vi "get channels.vi"(11 "EthernetIP configuration in":refnum<class "EIP Tags Configuration.lvclass">) -> (2 "channels":refnum<class "TBM channel.lvclass">[](array[class]), 3 "EthernetIP configuration out":refnum<class "EIP Tags Configuration.lvclass">)   [LabVIEW 2013, in "EIP Tags Configuration.lvclass"]
uses:
  EIP Tags Configuration.lvclass
  <vilib>/NI/Tag Bus Module Framework/channel/TBM channel.lvclass
  EIP Tags Configuration.lvclass/EIP Tags Configuration.ctl
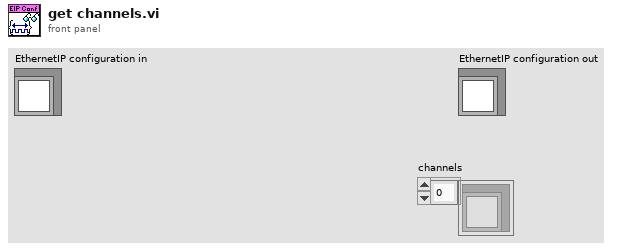
[diagram p1: front panel]
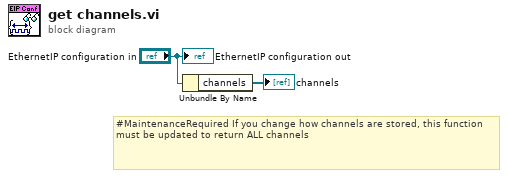
[diagram p0: block diagram]
diagram:
  # "#MaintenanceRequired If you change how channels are stored, this function must be updated to return ALL channels"
  n1 = Unbundle By Name("EthernetIP configuration in") -> ("channels"=→"channels":refnum<class "EIP Tags Channel.lvclass">[])
  "EthernetIP configuration out" <- "EthernetIP configuration in"
